vi "Keithley 6517 Perform Advance Triggering Setup.vi"() -> ()   [LabVIEW 2020]
doc: "This example shows how to bypass Measure Layer, Scan Layer or Arm Layer while the trigger source is trigger link and bypass is enabled.\n\n\n<B>Note:</B>\nThis Example is ONLY compatible with model 6517."
uses:
  <instrlib>/Keithley 6517/Keithley 6517.lvlib
panel:
  in  "Initiation Option (0: Immediate)":i32(ring) items=["Immediate", "Continuous"]
  in  "Bypass Option (0: Immediate)":i32(ring) items=["Immediate", "Signal"]
  in  "Output Trigger Line (2: Line2)":i32(ring)=2 items=["Line1"=1, "Line2"=2, "Line3"=3, "Line4"=4, "Line5"=5, "Line6"=6]
  in  "Input Trigger Line(1: Line1)":i32(ring)=1 items=["Line1"=1, "Line2"=2, "Line3"=3, "Line4"=4, "Line5"=5, "Line6"=6]
  in  "Triggers(0: Measure Layer)":u16(ring) items=["Measure Layer", "Scan Layer", "Arm Layer"]
  in  "VISA resource name":refnum<visa-resource-name>
  # "(c) 2016-2017 National Instruments.  ALL RIGHTS RESERVED."
  # "Note: This Example is ONLY compatible with model 6517."
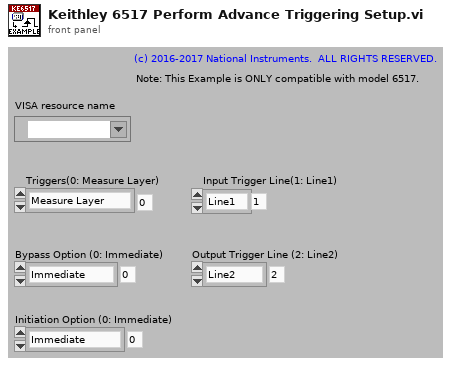
[diagram p1: front panel]
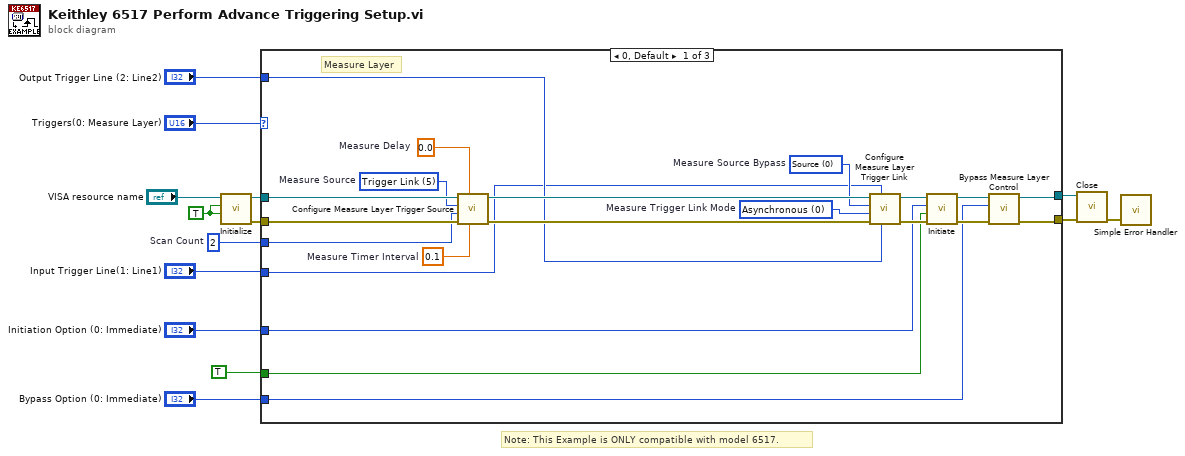
[diagram p0: block diagram]
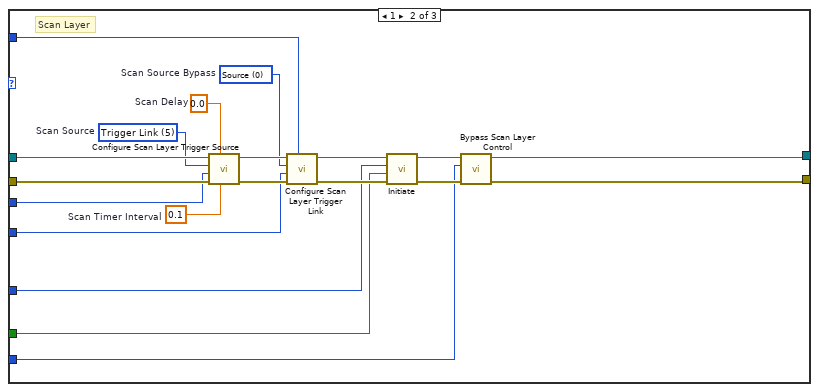
[diagram p2: hidden frame]
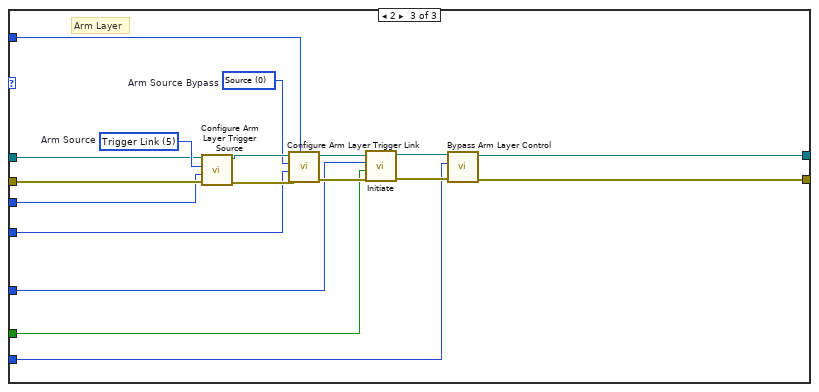
[diagram p3: hidden frame]
diagram:
  w2 = 2  # Scan Count
  w13 = TRUE ("ID Query (True)")
  # "Note: This Example is ONLY compatible with model 6517."
  n1 = call <instrlib>:"Initialize.vi"("Reset (True)"=w13, "ID Query (True)"=w13, "VISA resource name"="VISA resource name") -> ("error out"=w10:errorcluster, "VISA resource name out"=w11:refnum<visa-resource-name>)  [unwired: 7 in]
  n2 = case shown="0, Default" "Triggers(0: Measure Layer)" {
    tunnel: w11 -> [w35 w55 w65]
    tunnel: w10 -> [w34 w54 w64]
    tunnel: [w28 w47 w63] -> w9
    tunnel: [w27 w46 w62] -> w8
    tunnel: TRUE ("Include No-operation-pending Flag (T: Include No-operation-pending Flag)") -> [w23 w44 w61]
    tunnel: "Initiation Option (0: Immediate)" -> [w24 w45 w60]
    tunnel: "Output Trigger Line (2: Line2)" -> [w20 w42 w59]
    tunnel: "Input Trigger Line(1: Line1)" -> [w19 w40 w58]
    tunnel: "Bypass Option (0: Immediate)" -> [w22 w43 w57]
    tunnel: w2 -> [w15 w36 w56]
    frame 0, Default {
      w16 = 0.1  # Measure Timer Interval
      w17 = 0.0  # Measure Delay
      w18 = 0 items=["Asynchronous", "Synchronous"]  # Measure Trigger Link Mode
      w21 = 0 items=["Source", "Acceptor"]  # Measure Source Bypass
      w25 = 5 items=["Hold"=0, "Immediate"=1, "Manual"=3, "Bus"=4, "Trigger Link"=5, "External Triggering"=6, "Timer "=7]  # Measure Source
      # "Measure Layer"
      n3 = call <instrlib>:"Configure Measure Layer Trigger Source.vi"("Measure Timer Interval (0.1)"=w16, "Measure Delay (0 s)"=w17, "error in (no error)"=w34, "Measure Count (1)"=w15, "Measure Source (1: Immediate)"=w25, "VISA resource name"=w35) -> ("error out"=w32:errorcluster, "VISA resource name out"=w33:refnum<visa-resource-name>)  [unwired: 4 in]
      n4 = call <instrlib>:"Configure Measure Layer Trigger Link.vi"("Measure Output Trigger Line (1: Line1)"=w20, "Measure Input Trigger Line (2: Line2)"=w19, "error in (no error)"=w32, "Measure Trigger Link Mode (0: Asynchronous)"=w18, "Measure Source Bypass (1: Acceptor)"=w21, "VISA resource name"=w33) -> ("error out"=w30:errorcluster, "VISA resource name out"=w31:refnum<visa-resource-name>)  [unwired: 4 in]
      n5 = call <instrlib>:"Initiate.vi"("error in (no error)"=w30, "Include No-operation-pending Flag (True)"=w23, "Initiation Option (0: Immediate)"=w24, "VISA resource name"=w31) -> ("error out"=w26:errorcluster, "VISA resource name out"=w29:refnum<visa-resource-name>)  [unwired: 6 in]
      n6 = call <instrlib>:"Bypass Measure Layer Control.vi"("error in (no error)"=w26, "Measure Bypass Option (0: Immediate)"=w22, "VISA resource name"=w29) -> ("error out"=w27:errorcluster, "VISA resource name out"=w28:refnum<visa-resource-name>)  [unwired: 7 in]
    }
    frame 1 {
      w37 = 0.0  # Scan Delay
      w38 = 0.1  # Scan Timer Interval
      w39 = 5 items=["Hold"=0, "Immediate"=1, "Manual"=3, "Bus"=4, "Trigger Link"=5, "External Triggering"=6, "Timer "=7]  # Scan Source
      w41 = 0 items=["Source", "Acceptor"]  # Scan Source Bypass
      # "Scan Layer"
      n7 = call <instrlib>:"Configure Scan Layer Trigger Source.vi"("Scan Timer Interval (0.1)"=w38, "Scan Delay (0 s)"=w37, "error in (no error)"=w54, "Scan Count (1)"=w36, "Scan Source (1: Immediate)"=w39, "VISA resource name"=w55) -> ("error out"=w52:errorcluster, "VISA resource name out"=w53:refnum<visa-resource-name>)  [unwired: 4 in]
      n8 = call <instrlib>:"Configure Scan Layer Trigger Link.vi"("Scan Output Trigger Line (2: Line2)"=w42, "error in (no error)"=w52, "Scan Input Trigger Line (1: Line1)"=w40, "Scan Source Bypass (1: Acceptor)"=w41, "VISA resource name"=w53) -> ("error out"=w50:errorcluster, "VISA resource name out"=w51:refnum<visa-resource-name>)  [unwired: 5 in]
      n9 = call <instrlib>:"Initiate.vi"("error in (no error)"=w50, "Include No-operation-pending Flag (True)"=w44, "Initiation Option (0: Immediate)"=w45, "VISA resource name"=w51) -> ("error out"=w48:errorcluster, "VISA resource name out"=w49:refnum<visa-resource-name>)  [unwired: 6 in]
      n10 = call <instrlib>:"Bypass Scan Layer Control.vi"("error in (no error)"=w48, "Scan Bypass Option (0: Immediate)"=w43, "VISA resource name"=w49) -> ("error out"=w46:errorcluster, "VISA resource name out"=w47:refnum<visa-resource-name>)  [unwired: 7 in]
    }
    frame 2 {
      w67 = 0 items=["Source", "Acceptor"]  # Arm Source Bypass
      w66 = 5 items=["Hold", "Immediate", "Real-time Clock", "Manual", "Bus", "Trigger Link", "External Triggering"]  # Arm Source
      # "Arm Layer"
      n11 = call <instrlib>:"Configure Arm Layer Trigger Source.vi"("error in (no error)"=w64, "Arm Count (1)"=w56, "Arm Source (1: Immediate)"=w66, "VISA resource name"=w65) -> ("error out"=w69:errorcluster, "VISA resource name out"=w68:refnum<visa-resource-name>)  [unwired: 6 in]
      n12 = call <instrlib>:"Configure Arm Layer Trigger Link.vi"("Arm Output Trigger Line (2: Line2)"=w59, "error in (no error)"=w69, "Arm Input Trigger Line (1: Line1)"=w58, "Arm Source Bypass (1: Acceptor)"=w67, "VISA resource name"=w68) -> ("error out"=w71:errorcluster, "VISA resource name out"=w70:refnum<visa-resource-name>)  [unwired: 5 in]
      n13 = call <instrlib>:"Initiate.vi"("error in (no error)"=w71, "Include No-operation-pending Flag (True)"=w61, "Initiation Option (0: Immediate)"=w60, "VISA resource name"=w70) -> ("error out"=w73:errorcluster, "VISA resource name out"=w72:refnum<visa-resource-name>)  [unwired: 6 in]
      n14 = call <instrlib>:"Bypass Arm Layer Control.vi"("error in (no error)"=w73, "Arm Bypass Option (0: Immediate)"=w57, "VISA resource name"=w72) -> ("error out"=w62:errorcluster, "VISA resource name out"=w63:refnum<visa-resource-name>)  [unwired: 7 in]
    }
  }
  n15 = call <instrlib>:"Close.vi"("error in (no error)"=w8, "VISA resource name"=w9) -> ("error out"=w1:errorcluster)  [unwired: 9 in]
  n16 = call <vilib>:"Simple Error Handler.vi"("error in (no error)"=w1) -> ()  [unwired: 4 in, 5 out]
